vi "FTW-CodeGen-FindGObjectTaggedForScripting.vi"(0 "GObject to Traverse":refnum<vi>, 5 "Class Name":string="GObject", 7 "Label Prefix to uniquely identify node":string="#FTW-CodeGen", 11 "error in":errorcluster) -> (6 "GObject":refnum<vi>, 15 "error out":errorcluster)   [LabVIEW 2013, in "FTW-CodeGen.lvlib"]
uses:
  FTW-CodeGen.lvlib
panel:
  # "Inputs"
  # "Outputs"
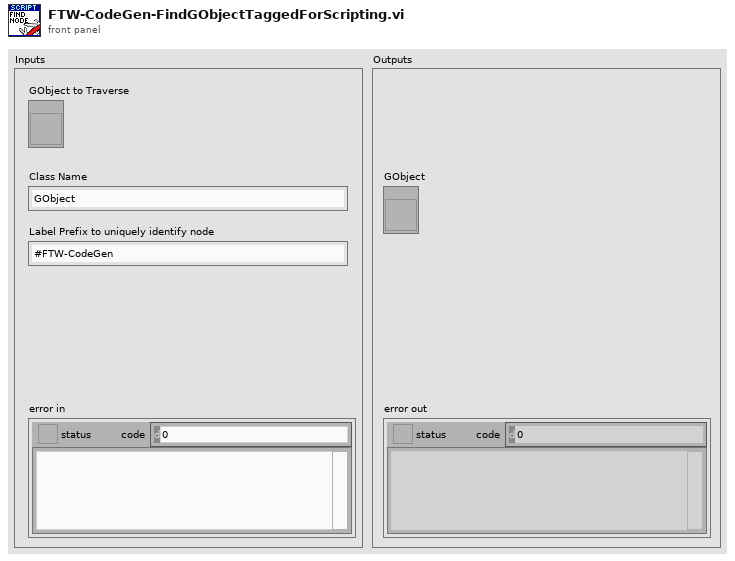
[diagram p1: front panel]
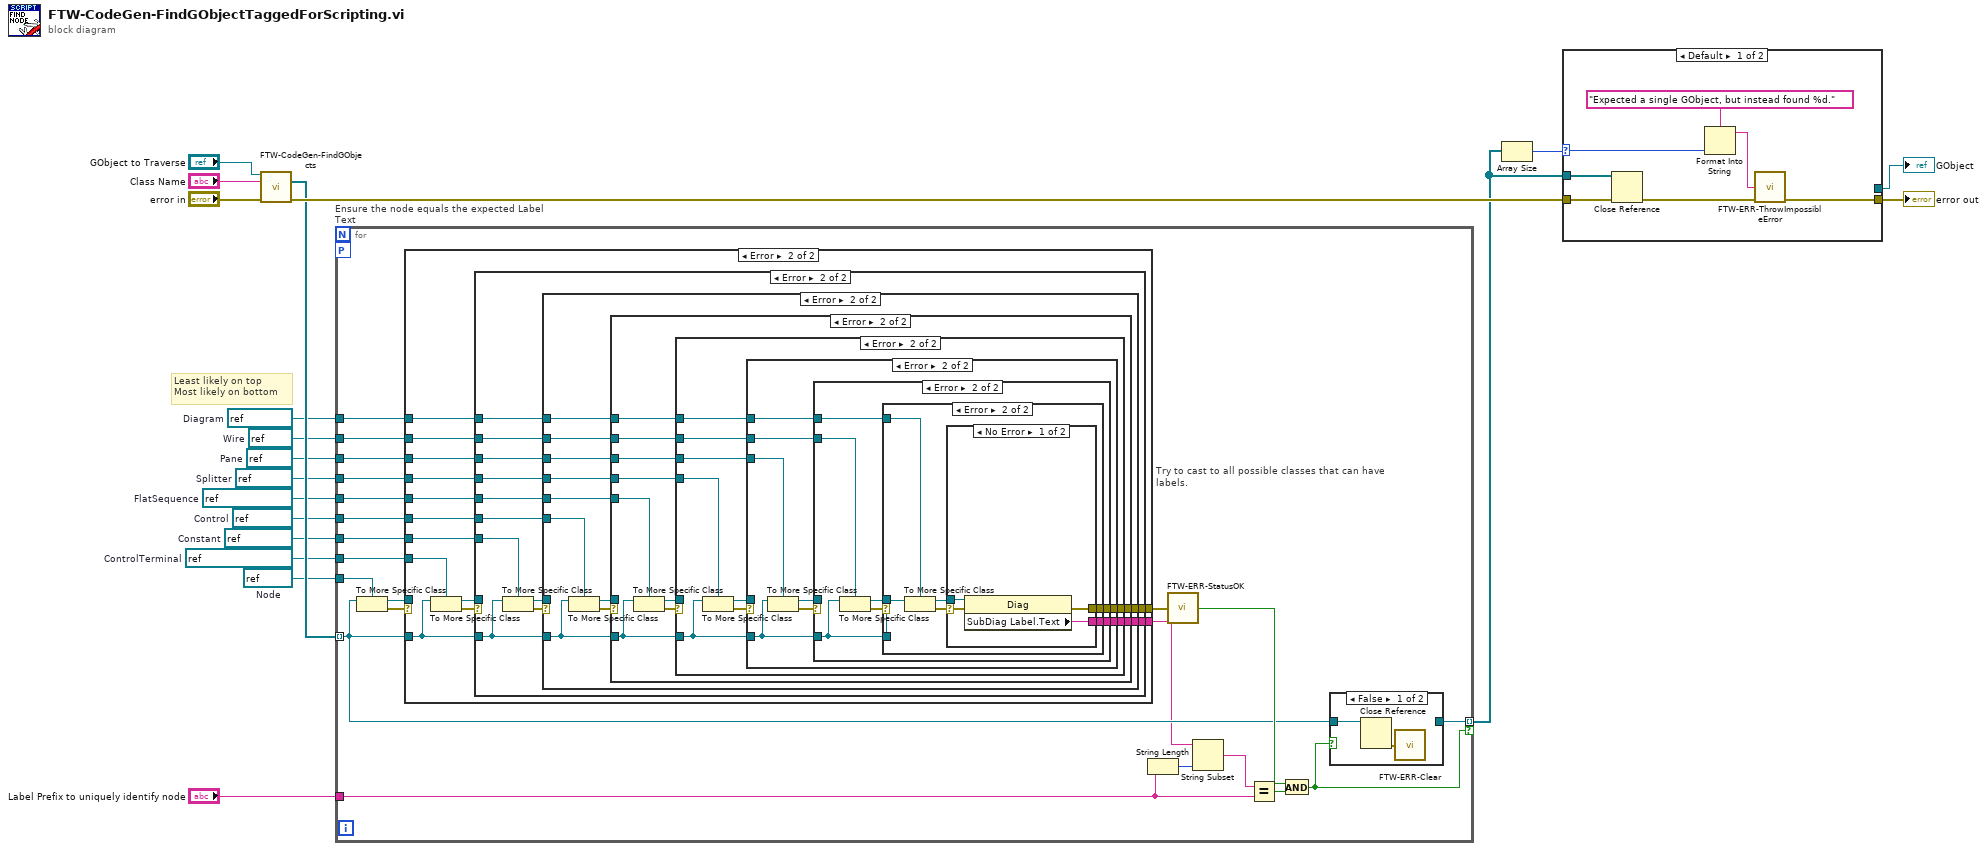
[diagram p0: block diagram]
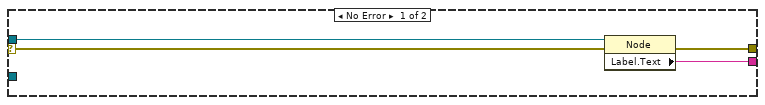
[diagram p3: hidden frame]
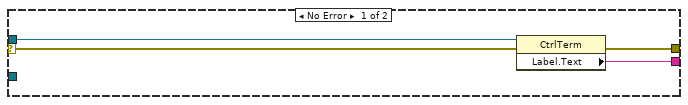
[diagram p4: hidden frame]
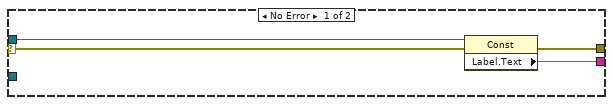
[diagram p5: hidden frame]
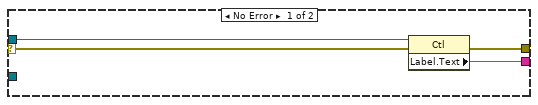
[diagram p6: hidden frame]
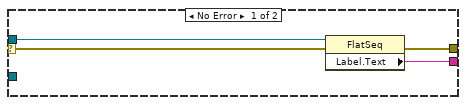
[diagram p7: hidden frame]
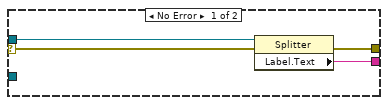
[diagram p8: hidden frame]
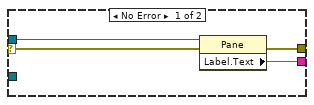
[diagram p9: hidden frame]
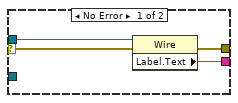
[diagram p10: hidden frame]
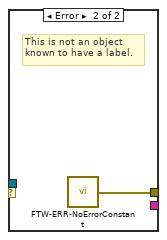
[diagram p11: hidden frame]
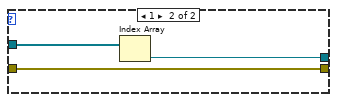
[diagram p12: hidden frame]
diagram:
  w3 = refnum<vi> refnum  # Constant
  w2 = refnum<vi> refnum  # ControlTerminal
  w4 = refnum<vi> refnum  # Control
  w5 = refnum<vi> refnum  # FlatSequence
  w6 = refnum<vi> refnum  # Splitter
  w7 = refnum<vi> refnum  # Pane
  w8 = refnum<vi> refnum  # Wire
  w9 = refnum<vi> refnum  # Diagram
  w1 = refnum<vi> refnum  # Node
  # "Least likely on top\nMost likely on bottom"
  n1 = call "FTW-CodeGen-FindGObjects.vi"("GObject to Traverse"="GObject to Traverse", "Class Name"="Class Name", "error in"="error in") -> ("GObject Instances"=w12:refnum<vi>[], "error out"=w14:errorcluster)  [unwired: 11 in]
  n2 = for "Ensure the node equals the expected Label Text" {
    tunnel: w12 -> [w26] mode=indexing
    tunnel: [w25] -> w11 mode=indexing if=w24
    workers-P: _ -> [_]
    tunnel: "Label Prefix to uniquely identify node" -> [w20]
    tunnel: w9 -> [w35]
    tunnel: w8 -> [w34]
    tunnel: w7 -> [w33]
    tunnel: w6 -> [w32]
    tunnel: w5 -> [w31]
    tunnel: w4 -> [w30]
    tunnel: w3 -> [w29]
    tunnel: w2 -> [w28]
    tunnel: w1 -> [w27]
    n3 = To More Specific Class(target class=w27, reference=w26) -> (specific class reference=w37:refnum<vi>, error out=w36:errorcluster)  [unwired: 1 in]
    n4 = case "Try to cast to all possible classes that can have labels." shown="Error" w36 {
      selector: w36 -> [w47 _]
      tunnel: w26 -> [_ w58]
      tunnel: w37 -> [w46 _]
      tunnel: [w45 w57] -> w38
      tunnel: [w44 w56] -> w23
      tunnel: w35 -> [_ w55]
      tunnel: w34 -> [_ w54]
      tunnel: w33 -> [_ w53]
      tunnel: w32 -> [_ w52]
      tunnel: w31 -> [_ w51]
      tunnel: w30 -> [_ w50]
      tunnel: w29 -> [_ w49]
      tunnel: w28 -> [_ w48]
      frame No Error {
        n5 = property class="Node"(reference=w46, error in=w47) -> (error out=w45:errorcluster, "Label.Text"=w44:string)  [unwired: 1 out]
      }
      frame Error {
        n6 = To More Specific Class(target class=w48, reference=w58) -> (specific class reference=w59:refnum<vi>, error out=w60:errorcluster)  [unwired: 1 in]
        n7 = case shown="Error" w60 {
          selector: w60 -> [w64 _]
          tunnel: w59 -> [w63 _]
          tunnel: w58 -> [_ w74]
          tunnel: [w62 w73] -> w57
          tunnel: [w61 w72] -> w56
          tunnel: w55 -> [_ w71]
          tunnel: w54 -> [_ w70]
          tunnel: w53 -> [_ w69]
          tunnel: w52 -> [_ w68]
          tunnel: w51 -> [_ w67]
          tunnel: w50 -> [_ w66]
          tunnel: w49 -> [_ w65]
          frame No Error {
            n8 = property class="CtrlTerm"(reference=w63, error in=w64) -> (error out=w62:errorcluster, "Label.Text"=w61:string)  [unwired: 1 out]
          }
          frame Error {
            n9 = To More Specific Class(target class=w65, reference=w74) -> (specific class reference=w75:refnum<vi>, error out=w76:errorcluster)  [unwired: 1 in]
            n10 = case shown="Error" w76 {
              selector: w76 -> [w80 _]
              tunnel: w75 -> [w79 _]
              tunnel: w74 -> [_ w89]
              tunnel: [w78 w88] -> w73
              tunnel: [w77 w87] -> w72
              tunnel: w71 -> [_ w86]
              tunnel: w70 -> [_ w85]
              tunnel: w69 -> [_ w84]
              tunnel: w68 -> [_ w83]
              tunnel: w67 -> [_ w82]
              tunnel: w66 -> [_ w81]
              frame No Error {
                n11 = property class="Const"(reference=w79, error in=w80) -> (error out=w78:errorcluster, "Label.Text"=w77:string)  [unwired: 1 out]
              }
              frame Error {
                n12 = To More Specific Class(target class=w81, reference=w89) -> (specific class reference=w90:refnum<vi>, error out=w91:errorcluster)  [unwired: 1 in]
                n13 = case shown="Error" w91 {
                  selector: w91 -> [w95 _]
                  tunnel: w90 -> [w94 _]
                  tunnel: w89 -> [_ w102]
                  tunnel: [w93 w103] -> w88
                  tunnel: [w92 w101] -> w87
                  tunnel: w86 -> [_ w100]
                  tunnel: w85 -> [_ w99]
                  tunnel: w84 -> [_ w98]
                  tunnel: w83 -> [_ w97]
                  tunnel: w82 -> [_ w96]
                  frame No Error {
                    n14 = property class="Ctl"(reference=w94, error in=w95) -> (error out=w93:errorcluster, "Label.Text"=w92:string)  [unwired: 1 out]
                  }
                  frame Error {
                    n15 = To More Specific Class(target class=w96, reference=w102) -> (specific class reference=w104:refnum<vi>, error out=w105:errorcluster)  [unwired: 1 in]
                    n16 = case shown="Error" w105 {
                      selector: w105 -> [w109 _]
                      tunnel: w104 -> [w108 _]
                      tunnel: [w107 w115] -> w103
                      tunnel: w102 -> [_ w117]
                      tunnel: [w106 w114] -> w101
                      tunnel: w100 -> [_ w113]
                      tunnel: w99 -> [_ w112]
                      tunnel: w98 -> [_ w111]
                      tunnel: w97 -> [_ w110]
                      frame No Error {
                        n17 = property class="FlatSeq"(reference=w108, error in=w109) -> (error out=w107:errorcluster, "Label.Text"=w106:string)  [unwired: 1 out]
                      }
                      frame Error {
                        n18 = To More Specific Class(target class=w110, reference=w117) -> (specific class reference=w116:refnum<vi>, error out=w118:errorcluster)  [unwired: 1 in]
                        n19 = case shown="Error" w118 {
                          selector: w118 -> [w120 _]
                          tunnel: w117 -> [_ w126]
                          tunnel: w116 -> [w122 _]
                          tunnel: [w121 w129] -> w115
                          tunnel: [w119 w127] -> w114
                          tunnel: w113 -> [_ w125]
                          tunnel: w112 -> [_ w124]
                          tunnel: w111 -> [_ w123]
                          frame No Error {
                            n20 = property class="Splitter"(reference=w122, error in=w120) -> (error out=w121:errorcluster, "Label.Text"=w119:string)  [unwired: 1 out]
                          }
                          frame Error {
                            n21 = To More Specific Class(target class=w123, reference=w126) -> (specific class reference=w128:refnum<vi>, error out=w130:errorcluster)  [unwired: 1 in]
                            n22 = case shown="Error" w130 {
                              selector: w130 -> [w134 _]
                              tunnel: [w132 w138] -> w129
                              tunnel: w128 -> [w133 _]
                              tunnel: [w131 w141] -> w127
                              tunnel: w126 -> [_ w137]
                              tunnel: w125 -> [_ w136]
                              tunnel: w124 -> [_ w135]
                              frame No Error {
                                n23 = property class="Pane"(reference=w133, error in=w134) -> (error out=w132:errorcluster, "Label.Text"=w131:string)  [unwired: 1 out]
                              }
                              frame Error {
                                n24 = To More Specific Class(target class=w135, reference=w137) -> (specific class reference=w139:refnum<vi>, error out=w140:errorcluster)  [unwired: 1 in]
                                n25 = case shown="Error" w140 {
                                selector: w140 -> [w144 _]
                                tunnel: [w142 w151] -> w141
                                tunnel: w139 -> [w145 _]
                                tunnel: [w143 w147] -> w138
                                tunnel: w137 -> [_ w150]
                                tunnel: w136 -> [_ w146]
                                frame No Error {
                                n26 = property class="Wire"(reference=w145, error in=w144) -> (error out=w143:errorcluster, "Label.Text"=w142:string)  [unwired: 1 out]
                                }
                                frame Error {
                                n27 = To More Specific Class(target class=w146, reference=w150) -> (specific class reference=w148:refnum<vi>, error out=w149:errorcluster)  [unwired: 1 in]
                                n28 = case shown="No Error" w149 {
                                selector: w149 -> [w152 _]
                                tunnel: [w153 _] -> w151
                                tunnel: w148 -> [w155 _]
                                tunnel: [w154 w156] -> w147
                                frame No Error {
                                n29 = property class="Diag"(reference=w155, error in=w152) -> (error out=w154:errorcluster, "SubDiag Label.Text"=w153:string)  [unwired: 1 out]
                                }
                                frame Error {
                                # "This is not an object\nknown to have a label."
                                n30 = call "FTW-ERR-NoErrorConstant.vi"() -> ("no error"=w156:errorcluster)
                                }
                                }
                                }
                                }
                              }
                            }
                          }
                        }
                      }
                    }
                  }
                }
              }
            }
          }
        }
      }
    }
    n31 = String Length(string=w20) -> (length=w21:i32)
    n32 = call "FTW-ERR-StatusOK.vi"("error to check"=w38) -> ("Status OK?"=w40:bool)
    n33 = String Subset(string=w23, length (rest)=w21) -> (substring=w22:string)  [unwired: 1 in]
    n34 = Equal?(x=w22, y=w20) -> (x = y?=w39:bool)
    n35 = And(x=w40, y=w39) -> (x .and. y?=w24:bool)
    n36 = case shown="False" w24 {
      tunnel: [_ w43] -> w25
      tunnel: w26 -> [w42 w43]
      frame False {
        n37 = Close Reference(reference=w42) -> (error out=w41:errorcluster)  [unwired: 1 in]
        n38 = call "FTW-ERR-Clear.vi"("error to snuff"=w41) -> ()  [unwired: 1 out]
      }
      frame True {
      }
    }
  }
  n39 = Array Size(array=w11) -> (size(s)=w16:i32)
  n40 = case shown="Default" w16 {
    selector: w16 -> [w161 _]
    tunnel: [w163 w166] -> w15
    tunnel: w14 -> [w158 w166]
    tunnel: w11 -> [w159 w165]
    tunnel: [_ w164] -> w13
    frame Default {
      n41 = Close Reference(reference=w159, error in (no error)=w158) -> (error out=w157:errorcluster)
      n42 = Format Into String(format string="Expected a single GObject, but instead found %d." ("Reason this error should never happen"), w161) -> (resulting string=w160:string)  [unwired: 2 in, 1 out]
      n43 = call "FTW-ERR-ThrowImpossibleError.vi"("Reason this error should never happen"=w160, "error in"=w157) -> ("error out"=w163:errorcluster)  [unwired: 13 in]
    }
    frame 1 {
      n44 = Index Array(array=w165) -> (element=w164:refnum<vi>)  [unwired: 1 in]
    }
  }
  "error out" <- w15
  "GObject" <- w13
